vi "HFRR ADV v02.vi"() -> ()   [LabVIEW 2025] (continued)
    frame Disabled {
      n3597 = case shown="True" {
        selector: _ -> [_ _]
        tunnel: w4745 -> [_ w4746]
        frame False {
        }
        frame True {
          n3598 = while {
            tunnel: [w4752] -> _
            tunnel: w4746 -> [_]
            i -> [w4752]
            stop <- w4747 stop-if-true
            n3599 = local read "Json End Flg"() -> (w4751:bool)
            n3600 = Wait (ms)(milliseconds to wait=u32 20 ("Refresh Rate (ms)")) -> ()  [unwired: 1 out]
            n3601 = local read "refresh flag"() -> (w4748:bool)
            n3602 = local read "RUN"() -> (w4749:bool)
            n3603 = And(x=w4749, y=w4748) -> (x .and. y?=w4750:bool)
            n3604 = Or(x=w4750, y=w4751) -> (x .or. y?=w4753:bool)
            "AR Led" <- w4753
            n3605 = case shown="True" w4753 {
              frame False {
              }
              frame True {
                w4770 = "\",\""
                n3606 = local read "UUID"() -> (w4768:string)
                n3607 = local write "refresh flag"(FALSE ("refresh flag")) -> ()
                n3608 = local read "time"() -> (w4757:dbl)
                n3609 = Multiply(x=w4757, y=60.0) -> (x*y=w4756:dbl)
                n3610 = Concatenate Strings("UUID\" : \"", w4768, "\"}") -> (w4771:string)
                n3611 = Number To Fractional String(number=w4756, width (-)=i16 10, precision (6)=i16 4) -> (F-format string=w4785:string)  [unwired: 1 in]
                n3612 = Concatenate Strings("{", "\"Time\":\"", w4785, w4770) -> (w4780:string)
                n3613 = stacked-sequence {
                  tunnel: w4770 -> [w4833 w4841 w4848 w4856 w4864 w4873 w4880]
                  tunnel: [w4834 _ _ _ _ _ _] -> w4784
                  tunnel: [_ w4842 _ _ _ _ _] -> w4783
                  tunnel: [_ _ w4849 _ _ _ _] -> w4782
                  tunnel: [_ _ _ w4858 _ _ _] -> w4781
                  tunnel: w4771 -> [_ _ _ _ _ _ w4891]
                  tunnel: [_ _ _ _ _ _ w4890] -> w4767
                  tunnel: [_ _ _ _ _ w4870 _] -> w4766
                  tunnel: [_ _ _ _ w4863 _ _] -> w4765
                  frame #0 {
                    n3614 = local read "NORMAL LOAD"() -> (w4832:dbl)
                    n3615 = Number To Fractional String(number=w4832, width (-)=i16 10, precision (6)=i16 4) -> (F-format string=w4835:string)  [unwired: 1 in]
                    n3616 = Concatenate Strings("NormalLoad\":\"", w4835, w4833) -> (w4834:string)
                  }
                  frame #1 {
                    n3617 = local read "Temp"() -> (w4840:dbl)
                    n3618 = Number To Fractional String(number=w4840, width (-)=i16 10, precision (6)=i16 4) -> (F-format string=w4843:string)  [unwired: 1 in]
                    n3619 = Concatenate Strings("Temperature\":\"", w4843, w4841) -> (w4842:string)
                  }
                  frame #2 {
                    n3620 = local read "cof"() -> (w4846:dbl)
                    n3621 = Number To Fractional String(number=w4846, width (-)=i16 10, precision (6)=i16 4) -> (F-format string=w4850:string)  [unwired: 1 in]
                    n3622 = Concatenate Strings("FrictionalForce\":\"", w4850, w4848) -> (w4849:string)
                  }
                  frame #3 {
                    n3623 = local read "Set Hz"() -> (w4854:dbl)
                    n3624 = Multiply(x=w4854, y=60.0) -> (x*y=w4853:dbl)
                    n3625 = Number To Fractional String(number=w4853, width (-)=i16 10, precision (6)=i16 4) -> (F-format string=w4859:string)  [unwired: 1 in]
                    n3626 = Concatenate Strings("Speed\":\"", w4859, w4856) -> (w4858:string)
                  }
                  frame #4 {
                    n3627 = local read item#-1() -> (w4862)
                    n3628 = Number To Fractional String(number=w4862, width (-)=i16 10, precision (6)=i16 4) -> (F-format string=w4866:string)  [unwired: 1 in]
                    n3629 = Concatenate Strings("LinearDeformation\":\"", w4866, w4864) -> (w4863:string)
                  }
                  frame #5 {
                    n3630 = local read "AIR TEMP"() -> (w4869:dbl)
                    n3631 = local read "Json St Flg"() -> (w4871:bool)
                    n3632 = local read "Json End Flg"() -> (w4872:bool)
                    n3633 = Number To Fractional String(number=w4869, width (-)=i16 10, precision (6)=i16 4) -> (F-format string=w4875:string)  [unwired: 1 in]
                    n3634 = Concatenate Strings("Vibration\":\"", w4875, w4873) -> (w4870:string)
                    n3635 = And(x=w4871, y=w4872) -> ()  [unwired: 1 out]
                  }
                  frame #6 {
                    n3636 = local read "Json End Flg"() -> (w4879:bool)
                    n3637 = Get Date/Time In Seconds() -> (seconds since 1Jan1904=w4887:timestamp)
                    n3638 = local read "Json St Flg"() -> (w4878:bool)
                    n3639 = To Double Precision Float(number=w4887) -> (double precision float=w4886:dbl)
                    n3640 = Subtract(x=w4886, y=2082844800.0) -> (x-y=w4884:dbl)
                    n3641 = Number To Fractional String(number=w4884, width (-)=i16 12, precision (6)=i16 0) -> (F-format string=w4881:string)  [unwired: 1 in]
                    n3642 = case shown="True" w4879 {
                      tunnel: ["" w4894] -> w4888
                      tunnel: w4881 -> [_ w4895]
                      tunnel: w4880 -> [_ w4893]
                      frame False {
                      }
                      frame True {
                        n3643 = local write "Json End Flg"(FALSE ("Json St Flg")) -> ()
                        n3644 = Concatenate Strings("End\": \"", w4895, w4893) -> (w4894:string)
                      }
                    }
                    n3645 = case shown="True" w4878 {
                      tunnel: [w4898 w4901] -> w4889
                      tunnel: w4881 -> [_ w4902]
                      tunnel: w4880 -> [_ w4899]
                      frame False {
                        n3646 = local read "St Str"() -> (w4898:string)
                      }
                      frame True {
                        n3647 = Concatenate Strings("Start\":\"", w4902, w4899) -> (w4901:string)
                        "St Str" <- w4901
                        n3648 = local write "Json St Flg"(FALSE ("Json St Flg")) -> ()
                      }
                    }
                    n3649 = Concatenate Strings(w4889, w4888, w4891) -> (w4890:string)
                  }
                }
                n3650 = local read "FILE"() -> (w4759:string)
                n3651 = Concatenate Strings("\",\"OperatorID\":\"" ("string"), "Operator ID") -> (w4762:string)
                n3652 = Concatenate Strings("\",\"DatasetTitle\":\"" ("string"), w4759) -> (w4761:string)
                n3653 = Concatenate Strings("\",\"SerialNumber\":\"" ("string"), "Serial No") -> (w4791:string)
                n3654 = Concatenate Strings("\",\"ModelNumber\":\"" ("string"), "Model No") -> (w4790:string)
                n3655 = Concatenate Strings(w4791, w4790) -> (w4773:string)
                n3656 = Concatenate Strings("{\"SecretKey\":\"", "Secret Key", w4773, w4762, w4761, "\",\"Samples\":[") -> (w4778:string)
                n3657 = Concatenate Strings(w4780, w4784, w4783, w4782, w4781, w4765, w4766, w4767) -> (w4779:string)
                n3658 = Concatenate Strings(w4778, w4779, "]}") -> (w4777:string)
                n3659 = stacked-sequence {
                  tunnel: w4777 -> [w4806 _ _]
                  tunnel: [_ _ w4823] -> _
                  frame #0 {
                    (unwired) FALSE ("convert eol (F)")
                    w4808 = enum16{"start", "end", "current"}."start" ("pos mode (0:2)")
                    n3660 = Path To String(path="Path") -> (string=w4814:string)
                    n3661 = Concatenate Strings(w4814, "\\", "Data File Name") -> (w4816:string)
                    n3662 = local write "standard output"(" ") -> ()
                    n3663 = String To Path(string=w4816) -> (path=w4805:path)
                    n3664 = call <vilib>:"Open_Create_Replace File.vi"("advisory dialog? (display:T)"=FALSE, "function (open:0)"=T25."create or replace", "file path"=w4805) -> ("error out"=w4819:errorcluster, "refnum"=w4818:refnum<file>)  [unwired: 5 in, 2 out]
                    n3665 = Set File Position(refnum=w4818, from (0:start)=w4808, error in=w4819) -> (refnum out=w4799:refnum<file>, error out=w4798:errorcluster)  [unwired: 1 in]
                    n3666 = Write to Binary File(file (use dialog)=w4799, data=" ", error in=w4798, 5:FALSE ("prepend array or string size? (T)")) -> (refnum out=w4809:refnum<file>, error out=w4810:errorcluster)  [unwired: 2 in, 1 out]
                    n3667 = Set File Position(offset (in bytes) (0)=w4808, refnum=w4809, error in=w4810) -> (refnum out=w4802:refnum<file>, error out=w4801:errorcluster)  [unwired: 1 in]
                    n3668 = Write to Binary File(file (use dialog)=w4802, data=w4806, error in=w4801, 5:FALSE ("prepend array or string size? (T)")) -> (error out=w4804:errorcluster)  [unwired: 2 in, 2 out]
                    n3669 = flat-sequence {
                      tunnel: w4805 -> [w4821]
                      tunnel: w4804 -> [_]
                      frame #0 {
                        n3670 = call <vilib>:"Read Characters From File.vi"("file path (dialog if empty)"=w4821) -> ("character string"=→"JSON string":string)  [unwired: 5 in, 3 out]
                      }
                    }
                    "SinglePoint" <- w4806
                  }
                  frame #1 {
                  }
                  frame #2 {
                    (unwired) "\"Stored\": true" ("string")
                    n3671 = call <vilib>:"System Exec.vi"("run minimized? (F)"=TRUE, "wait until completion? (T)"=TRUE, "working directory"=path "C:/LAB-IQ-NXT", "command line"="C:\\LAB-IQ-NXT\\JPost.bat") -> ("standard error"=→"Respose From Server":string, "standard output"=w4826:string)  [unwired: 4 in, 2 out]
                    "standard output" <- w4826
                    n3672 = Match Pattern(string=w4826, regular expression="JSON Check String") -> (match substring=w4824:string, offset past match=w4823:i32)  [unwired: 1 in, 2 out]
                    n3673 = Equal?(x=w4824, y="JSON Check String") -> (x = y?=→"Upload \nConfirmed":bool)
                  }
                }
              }
            }
            n3674 = local read "Quit"() -> (w4747:bool)
          }
        }
      }
    }
    frame Enabled {
    }
  }
  n3675 = disable-structure shown="Disabled" {
    disable-tunnel: _ -> [w4909 _]
    frame Disabled {
      n3676 = while {
        shift-right: [w4917] -> w4905
        shift-left: _ -> [w4918]
        shift-right: [w4915] -> w4906
        shift-left: errorcluster {"status"=TRUE, "code"=0, "source"="Init"} ("error out") -> [w4916]
        shift-right: [w4913] -> _
        shift-left: "" -> [w4914]
        tunnel: [w4911] -> _
        tunnel: w4909 -> [_]
        i -> [w4911]
        stop <- w4910 stop-if-true
        n3677 = flat-sequence {
          tunnel: [w4919] -> w4912
          frame #0 {
            n3678 = Wait (ms)(milliseconds to wait=10.0 ("Delay")) -> (millisecond timer value=w4919:u32)
          }
        }
        n3679 = case shown="No Error" w4916 {
          selector: w4916 -> [w4949 w5068]
          tunnel: [w4932 w5070] -> w4917
          tunnel: [w4931 w5069] -> w4915
          tunnel: w4918 -> [w4950 w5062]
          tunnel: w4914 -> [w4930 w5061]
          tunnel: [w4929 w5061] -> w4913
          tunnel: w4912 -> [_ _]
          frame No Error {
            n3680 = Concatenate Strings("\r", "\n") -> (w4941:string)  [unwired: 1 in]
            n3681 = case shown="True" w4942 {
              tunnel: w4950 -> [w4974 w4981]
              tunnel: w4949 -> [w4973 w4980]
              tunnel: [w4974 w4979] -> w4948
              tunnel: [w4973 w4978] -> w4928
              tunnel: w4941 -> [_ w4977]
              frame False {
              }
              frame True {
                n3682 = VISA Write(VISA resource name=w4981, write buffer=w4977, error in (no error)=w4980) -> (VISA resource name out=w4979:refnum<visa-resource-name>, error out=w4978:errorcluster)  [unwired: 1 out]
                n3683 = local write "Read String"("") -> ()
                n3684 = local write item#-1(FALSE) -> ()
              }
            }
            n3685 = property class="Instr"(reference=w4948, error in=w4928) -> (reference out=w4947:refnum<visa-resource-name>, error out=w4946:errorcluster, "Serial Settings:Number of Bytes at Serial Port"=w4945:u32)
            n3686 = Greater?(x=w4945, y=u32 100) -> (0:w4943:bool)
            n3687 = case shown="True" w4943 {
              tunnel: w4947 -> [w4984 w5008]
              tunnel: w4946 -> [w4983 w5007]
              tunnel: w4945 -> [_ w5006]
              tunnel: [w4984 w5005] -> w4934
              tunnel: [w4983 w5004] -> w4933
              tunnel: w4930 -> [w4982 w5003]
              tunnel: [w4982 ""] -> w4929
              frame False {
              }
              frame True {
                w4993 = u32 6 ("y")
                # "Page 84 of \nmanual"
                n3688 = VISA Read(VISA resource name=w5008, byte count=w5006, error in (no error)=w5007) -> (VISA resource name out=w5005:refnum<visa-resource-name>, read buffer=w5001:string, error out=w5004:errorcluster)  [unwired: 1 out]
                n3689 = while {
                  tunnel: w5001 -> [w5057]
                  tunnel: [w5053] -> w4995 mode=indexing
                  tunnel: [w5047] -> w4999 mode=indexing
                  tunnel: [w5045] -> _
                  i -> [w5045]
                  stop <- w5050 stop-if-true
                  n3690 = String Subset(string=w5057, offset (0)=w5045) -> (substring=w5052:string)  [unwired: 1 in]
                  n3691 = String To Byte Array(string=w5052) -> (unsigned byte array=w5056:u8[])
                  n3692 = String Length(string=w5052) -> (length=w5051:i32)
                  n3693 = Index Array(array=w5056) -> (element=w5055:u8)  [unwired: 1 in]
                  n3694 = Equal To 0?(x=w5051) -> (x = 0?=w5050:bool)
                  n3695 = Number To Boolean Array(number=w5055) -> (Boolean array=w5049:bool[])
                  n3696 = Reverse 1D Array(array=w5049) -> (reversed array=w5048:bool[])
                  n3697 = And(x=w5049, y=bool[] [FALSE, FALSE, FALSE, FALSE, FALSE, FALSE, TRUE, TRUE] ("Boolean array")) -> (x .and. y?=w5053:bool[])
                  n3698 = And(x=w5048, y=bool[] [FALSE, FALSE, TRUE, TRUE, TRUE, TRUE, TRUE, TRUE] ("Boolean array")) -> (x .and. y?=w5047:bool[])
                }
                n3699 = Concatenate Strings(w5003, w5001) -> (→"Read String":string)
                n3700 = while {
                  tunnel: w4995 -> [w5044] mode=indexing
                  tunnel: [w5040] -> w4998
                  i -> [w5040]
                  stop <- w5041 stop-if-true
                  n3701 = Search 1D Array(1D array=w5044, element=TRUE) -> (index of element=w5042:i32)  [unwired: 1 in]
                  n3702 = Less Than 0?(x=w5042) -> (x < 0?=w5041:bool)
                }
                n3703 = Delete From Array(array=w4999, length=w4998, index (row)=0) -> (array with subset deleted=w4994:bool[][])  [unwired: 1 in, 1 out]
                n3704 = Array Size(array=w4994) -> (size(s)=w4996:i32[])
                n3705 = Index Array(array=w4996) -> (element=w4988:i32)  [unwired: 1 in]
                n3706 = Greater?(x=w4988, y=w4993) -> (0:w4991:bool)
                n3707 = Subtract(x=w4988, y=w4993) -> (x-y=w4992:u32)
                n3708 = Select(t=w4992, s=w4991, f=u32 0) -> (s? t:f=w4989:u32)
                n3709 = while {
                  tunnel: w4994 -> [w5027]
                  tunnel: [w5029] -> w4987 mode=indexing
                  tunnel: w4989 -> [w5011]
                  i -> [w5028]
                  stop <- w5026 stop-if-true
                  w5018 = 6 ("index")
                  w5017 = 2 ("length")
                  # "Page 65 of \nmanual"
                  n3710 = Multiply(x=u32 3 ("y"), y=w5028) -> (x*y=w5025:u32)
                  n3711 = Divide(x=u32 102 ("y"), y=u32 65520) -> (x/y=w5035:dbl)
                  n3712 = Greater Or Equal?(x=w5025, y=w5011) -> (x >= y?=w5026:bool)
                  n3713 = Index Array(array=w5027, index (row) #1=w5025) -> (element #1=w5023:bool[], element #2=w5022:bool[], element #3=w5021:bool[])  [unwired: 5 in]
                  n3714 = Reverse 1D Array(array=w5023) -> (reversed array=w5016:bool[])
                  n3715 = Reverse 1D Array(array=w5022) -> (reversed array=w5020:bool[])
                  n3716 = Reverse 1D Array(array=w5021) -> (reversed array=w5019:bool[])
                  n3717 = Delete From Array(array=w5016, length=w5017, index=w5018) -> (array with subset deleted=w5012:bool[])  [unwired: 1 out]
                  n3718 = Delete From Array(array=w5020, length=w5017, index=w5018) -> (array with subset deleted=w5013:bool[])  [unwired: 1 out]
                  n3719 = Delete From Array(array=w5019, length=w5017, index=w5018) -> (array with subset deleted=w5014:bool[])  [unwired: 1 out]
                  n3720 = Insert Into Array(array=bool[] [] ("Boolean array"), new element #1=w5012, new element #2=w5013, new element #3=w5014) -> (w5015:bool[])  [unwired: 1 in]
                  n3721 = Boolean Array To Number(Boolean array=w5015) -> (number=w5024:u32)
                  n3722 = Multiply(x=w5035, y=w5024) -> (x*y=w5034:dbl)
                  n3723 = Decrement(x=w5034) -> (x-1=w5033:dbl)
                  n3724 = Divide(x=w5033, y=u32 100) -> (x/y=w5031:dbl)
                  n3725 = Multiply(x=w5031, y=u32 10) -> (x*y=w5029:dbl)
                }
                n3726 = Delete From Array(array=w4987) -> (array with subset deleted=w4986:dbl[])  [unwired: 2 in, 1 out]
                "Waveform Graph 5" <- w4986
                "Waveform Chart 3" <- w4986
                n3727 = call-poly <vilib>:"Mean.vi"("X"=w4986) -> ("mean"=w4985:dbl)  [unwired: 1 out]
                n3728 = case shown="True" {
                  selector: _ -> [_ _]
                  tunnel: w4985 -> [_ w5010]
                  frame False {
                  }
                  frame True {
                    n3729 = local write item#-1(FALSE ("Zero 4")) -> ()
                    "z_measure" <- w5010
                  }
                }
              }
            }
            n3730 = local read item#-1() -> (w4925)
            n3731 = local read item#-1() -> (w4924)
            n3732 = local read item#-1() -> (w4926)
            n3733 = local read item#-1() -> (w4923)
            n3734 = case shown="True" w4921 {
              tunnel: w4925 -> [_ w4953]
              tunnel: w4926 -> [_ w4952]
              frame False {
              }
              frame True {
                n3735 = Build Array(w4953, w4952) -> (w4951:void[])
                n3736 = local read item#-1() -> (w4956)
                n3737 = Build Array (concatenate)(w4956, w4951) -> (w4954:void[])
                n3738 = local write item#-1(w4954) -> ()
                n3739 = local write item#-1(FALSE ("Boolean 8")) -> ()
              }
            }
            n3740 = call "Build XY Graph"("Enable"=w4923, "Reset"=w4924, "Y Input"=w4926, "X Input"=w4925) -> ("XY Graph"=w4922:cluster{"Y":dbl[], "Y":dbl[]}[])  [unwired: 6 in, 1 out]
            n3741 = case shown="True" {
              selector: _ -> [_ _]
              frame False {
              }
              frame True {
                n3742 = local read item#-1() -> (w4957)
                n3743 = Index Array(array=w4957, index (col) #1=0 ("disabled index (col)"), index (col) #2=1 ("index (col)")) -> (element #1=w4959, element #2=w4958)  [unwired: 2 in]
                n3744 = call <vilib>:"Linear Fit.vi"("Y"=w4959, "X"=w4958) -> ()  [unwired: 9 in, 5 out]
                n3745 = local write item#-1(FALSE ("Boolean 9")) -> ()
              }
            }
            n3746 = case shown="True" {
              selector: _ -> [_ _]
              frame False {
              }
              frame True {
                n3747 = local write item#-1(dbl[][] [] ("Captured Values")) -> ()
                n3748 = local write item#-1(FALSE ("Boolean 7")) -> ()
              }
            }
            n3749 = Concatenate Strings("\r", "\n") -> (w4936:string, w4935:string)
            n3750 = case shown="True" w4927 {
              tunnel: w4934 -> [w4966 w4972]
              tunnel: w4933 -> [w4965 w4971]
              tunnel: [w4966 w4970] -> w4932
              tunnel: [w4965 w4969] -> w4931
              tunnel: w4936 -> [_ w4968]
              frame False {
              }
              frame True {
                n3751 = VISA Write(VISA resource name=w4972, write buffer=w4968, error in (no error)=w4971) -> (VISA resource name out=w4970:refnum<visa-resource-name>, error out=w4969:errorcluster)  [unwired: 1 out]
                n3752 = local write item#-1(FALSE ("WRITE")) -> ()
              }
            }
          }
          frame Error {
            w5060 = u16 10 items=["1.0"=10, "1.5"=15, "2.0"=20] ("stop bits (10: 1 bit)")
            n3753 = Wait (ms)(milliseconds to wait=u32 20) -> ()  [unwired: 1 out]
            n3754 = VISA Close(VISA resource name=w5062, error in (no error)=w5068) -> (error out=w5067:errorcluster)
            n3755 = call <vilib>:"Clear Errors.vi"("error in (no error)"=w5067) -> ("error out"=w5066:errorcluster)  [unwired: 5 in, 1 out]
            n3756 = call-poly "VISA Configure Serial Port"("timeout (10sec)"=u32 200, "Enable Termination\nChar (T)"=TRUE ("Enable Termination\nChar (T)"), "baud rate (9600)"=u32 921600, "error in (no error)"=w5066, "stop bits (10: 1 bit)"=w5060) -> ("VISA resource name"=w5058:refnum<visa-resource-name>, "VISA resource name out"=w5070:refnum<visa-resource-name>, "error out"=w5069:errorcluster)  [unwired: 8 in]
          }
        }
        n3757 = local read "Quit"() -> (w4910:bool)
      }
      n3758 = VISA Close(VISA resource name=w4905, error in (no error)=w4906) -> (error out=w4904:errorcluster)
      n3759 = call <vilib>:"Clear Errors.vi"("error in (no error)"=w4904) -> ()  [unwired: 5 in, 2 out]
    }
    frame Enabled {
    }
  }
  n3760 = disable-structure shown="Disabled" {
    disable-tunnel: _ -> [w5075 _]
    frame Disabled {
      n3761 = while {
        tunnel: [w5082] -> _
        shift-right: [w5079] -> w5072
        shift-left: _ -> [w5081]
        shift-right: [w5080] -> w5073
        shift-left: errorcluster {"status"=TRUE, "code"=0, "source"="Init"} ("error out") -> [w5078]
        tunnel: w5075 -> [_]
        i -> [w5082]
        stop <- w5076 stop-if-true
        n3762 = flat-sequence {
          tunnel: w5078 -> [w5173]
          tunnel: [w5173] -> w5077
          frame #0 {
            n3763 = Wait (ms)(milliseconds to wait=u32 50) -> ()  [unwired: 1 out]
          }
        }
        n3764 = case shown="No Error" w5077 {
          selector: w5077 -> [w5123 w5166]
          tunnel: w5081 -> [w5122 w5165]
          tunnel: [w5089 w5156] -> w5080
          tunnel: [w5090 w5164] -> w5079
          frame No Error {
            w5116 = T26 {"Mode"=enum."RTU", "Slave Address"=1} ("Serial Parameters")
            n3765 = call-poly <vilib>:"MB Serial Master Query (poly).vi"("VISA resource name"=w5122, "Starting Address"=i16 1000, "Quantity"=u16 1, "Timeout"=u32 1000, "error in"=w5123, "Serial Parameters"=w5116) -> ("VISA resource name out"=w5117:refnum<visa-resource-name>, "Input Registers"=w5119:u16[], "error out"=w5115:errorcluster)  [unwired: 10 in, 1 out]
            n3766 = Random Number (0-1)() -> (number: 0 to 1=w5104:dbl)
            n3767 = Index Array(array=w5119, index=0) -> (element=w5114:u16)
            n3768 = Subtract(x=w5104, y=0.5) -> (x-y=w5103:dbl)
            n3769 = Divide(x=w5114, y=10 ("index")) -> (x/y=w5108:dbl)
            n3770 = Multiply(x=w5103, y=0.5) -> (x*y=w5102:dbl)
            n3771 = Add(x=w5108, y=w5102) -> (x+y=w5107:dbl)
            n3772 = local read "Amb temp"() -> (w5091:dbl)
            n3773 = Multiply(x=w5107, y=0.2) -> (x*y=w5111:dbl)
            n3774 = Multiply(x=w5091, y=0.8) -> (x*y=w5109:dbl)
            n3775 = Add(x=w5111, y=w5109) -> (x+y=w5092:dbl)
            n3776 = local read "set temp old"() -> (w5086:dbl)
            n3777 = local write "Amb temp"(w5092) -> ()
            n3778 = Select(t="SetTemp 2", s="Heater", f=100.0) -> (s? t:f=w5087:dbl)
            n3779 = Not Equal?(x=w5087, y=w5086) -> (x != y?=w5085:bool)
            n3780 = case shown="True" w5085 {
              tunnel: w5117 -> [w5151 w5153]
              tunnel: [w5150 w5153] -> w5097
              tunnel: w5115 -> [w5149 w5152]
              tunnel: [w5148 w5152] -> w5095
              tunnel: w5087 -> [w5143 _]
              tunnel: w5116 -> [w5145 w5154]
              tunnel: [w5145 w5154] -> w5098
              frame True {
                n3781 = Multiply(x=w5143, y=10 ("index")) -> (x*y=w5142:dbl)
                n3782 = call-poly <vilib>:"MB Serial Master Query (poly).vi"("VISA resource name"=w5151, "Address"=u16 0, "Holding Register"=w5142, "Timeout"=u32 1000, "error in"=w5149, "Serial Parameters"=w5145) -> ("VISA resource name out"=w5150:refnum<visa-resource-name>, "error out"=w5148:errorcluster)  [unwired: 11 in, 1 out]
                "set temp old" <- w5143
              }
              frame False {
              }
            }
            n3783 = flat-sequence {
              tunnel: [w5124] -> _
              tunnel: [w5124] -> w5094
              tunnel: w5095 -> [w5124]
              frame #0 {
                n3784 = Wait (ms)(milliseconds to wait=u32 100) -> ()  [unwired: 1 out]
              }
            }
            n3785 = call "Elapsed Time12"("Time Target (s)"=2.0, "Auto Reset"=TRUE) -> ("Time has Elapsed"=w5099:bool)  [unwired: 10 in, 7 out]
            n3786 = case shown="True" w5099 {
              tunnel: w5098 -> [w5128 w5141]
              tunnel: [w5128 w5141] -> _
              tunnel: [w5127 w5139] -> w5090
              tunnel: w5097 -> [w5127 w5140]
              tunnel: [w5126 w5137] -> w5089
              tunnel: w5094 -> [w5126 w5138]
              frame False {
              }
              frame True {
                n3787 = call-poly <vilib>:"MB Serial Master Query (poly).vi"("VISA resource name"=w5140, "Starting Address"=i16 1003 ("Addr"), "Quantity"=u16 1, "Timeout"=u32 1000, "error in"=w5138, "Serial Parameters"=w5141) -> ("VISA resource name out"=w5139:refnum<visa-resource-name>, "Input Registers"=w5134:u16[], "error out"=w5137:errorcluster)  [unwired: 10 in, 1 out]
                n3788 = Index Array(array=w5134, index=0) -> (element=w5133:u16)
                n3789 = Divide(x=w5133, y=u16 10) -> (x/y=w5129:dbl)
                n3790 = local write "set temp old"(w5129) -> ()
                n3791 = local write "SetTemp"(w5129) -> ()
              }
            }
            "Error Code" <- w5089
            n3792 = Unbundle(w5089) -> ("status"=→"TK4 status":bool)  [unwired: 2 out]
            "SetTemp" <- "SetTemp 2"
          }
          frame Error {
            w5168 = u16 0 items=["None", "Odd", "Even", "Mark", "Space"] ("Parity")
            w5169 = u16 0 items=["None", "XON/XOFF", "RTS/CTS", "XON/XOFF & RTS/CTS", "DTR/DSR", "XON/XOFF & DTR/DSR"] ("Flow Control")
            n3793 = VISA Clear(VISA resource name=w5165, error in (no error)=w5166) -> (VISA resource name out=w5159:refnum<visa-resource-name>, error out=w5157:errorcluster)
            n3794 = VISA Close(VISA resource name=w5159, error in (no error)=w5157) -> (error out=w5158:errorcluster)
            n3795 = call <vilib>:"Clear Errors.vi"("error in (no error)"=w5158) -> ("error out"=w5167:errorcluster)  [unwired: 5 in, 1 out]
            n3796 = Unbundle By Name(T26 {"Mode"=enum."RTU", "Slave Address"=1} ("input cluster")) -> ("Mode"=w5170:enum16{"RTU", "ASCII"})
            n3797 = call <vilib>:"MB Serial Init.vi"("Timeout"=u32 100, "Flow Control"=w5169, "Mode"=w5170, "error in (no error)"=w5167, "Parity"=w5168, "Baud Rate"=u32 9600, "VISA resource name"="Lubrication System COM Port :") -> ("error out"=w5156:errorcluster, "VISA resource name out"=w5164:refnum<visa-resource-name>)  [unwired: 3 in]
            n3798 = local write "set temp old"(0.0 ("set temp old")) -> ()
            n3799 = Unbundle(w5156) -> ("status"=w5155:bool)  [unwired: 2 out]
            n3800 = case shown="True" w5155 {
              selector: w5155 -> [_ w5172]
              frame False {
              }
              frame True {
                n3801 = local write "TK4 status"(w5172) -> ()
              }
            }
          }
        }
        n3802 = local read "Quit"() -> (w5076:bool)
      }
      n3803 = VISA Close(VISA resource name=w5072, error in (no error)=w5073) -> (error out=w5071:errorcluster)
      n3804 = call <vilib>:"Clear Errors.vi"("error in (no error)"=w5071) -> ()  [unwired: 5 in, 2 out]
    }
    frame Enabled {
    }
  }
